vi "Write Exception Status.vi"(8 "error in (no error)":errorcluster, 10 "exception status":u8 format="%02x", 11 "Modbus slave in":refnum<class "Modbus Slave.lvclass">) -> (0 "error out":errorcluster, 3 "Modbus slave out":refnum<class "Modbus Slave.lvclass">)   [LabVIEW 2021, in "Modbus Slave.lvclass"]
doc: "Writes the exception status of a Modbus slave. The exception status is a set of eight status bits. Each status bit represents an exception."
uses:
  Modbus Slave.lvclass
  Modbus Slave.lvclass/Modbus Slave.ctl
  Data Model/Device Data Model.lvclass
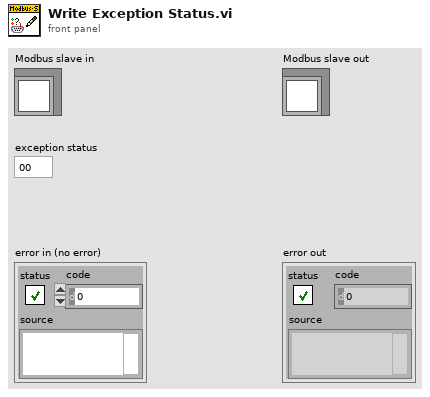
[diagram p1: front panel]
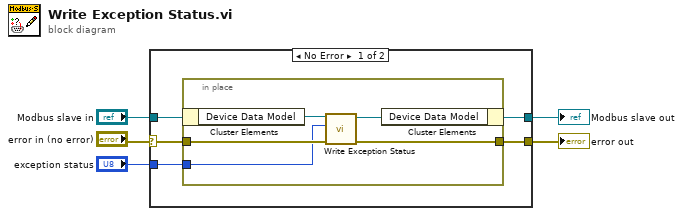
[diagram p0: block diagram]
diagram:
  n1 = case shown="No Error" "error in (no error)" {
    selector: "error in (no error)" -> [w8 w16]
    tunnel: "Modbus slave in" -> [w10 w17]
    tunnel: [w9 w17] -> w4
    tunnel: [w7 w16] -> w2
    tunnel: "exception status" -> [w6 _]
    frame No Error {
      n2 = in-place {
        in-place-border: w8 -> [w13]
        in-place-border: [w12] -> w7
        in-place-border: w6 -> [w11]
        n3 = in-place-cluster #1(w10) -> ("Device Data Model"=w15:refnum<class "Device Data Model.lvclass">)
        n4 = call-dynamic "Write Exception Status.vi"("error in"=w13, "exception status"=w11, "device data model in"=w15) -> ("error out"=w12:errorcluster, "device data model out"=w14:refnum<class "Device Data Model.lvclass">)  [unwired: 7 in]
        n5 = in-place-cluster #1("Device Data Model"=w14) -> (w9:refnum<class "Modbus Slave.lvclass">)
      }
    }
    frame Error {
    }
  }
  "Modbus slave out" <- w4
  "error out" <- w2
